vi "Destroy Subscription.vi"(8 "error in (no error)":errorcluster, 11 "Subscription in":refnum<class "Subscription.lvclass">) -> (0 "error out":errorcluster, 3 "Subscription out":refnum<class "Subscription.lvclass">)   [LabVIEW 2013, in "MQTT Server.lvlib" / "Subscription.lvclass"]
uses:
  Subscription.lvclass
  Subscription.lvclass/Subscription.ctl
  TopicFilter/TopicFilter.lvclass
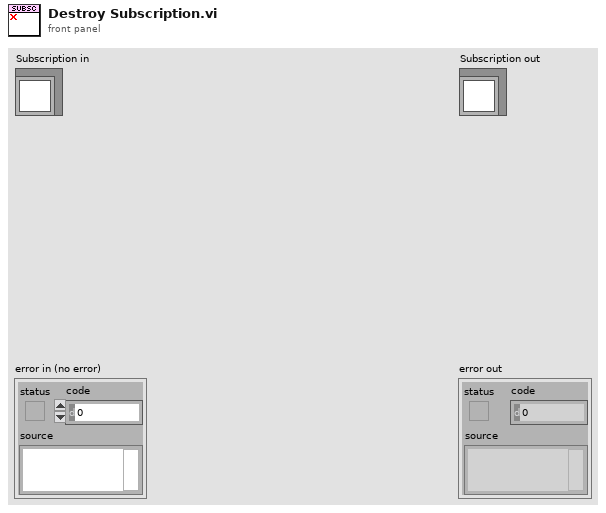
[diagram p1: front panel]
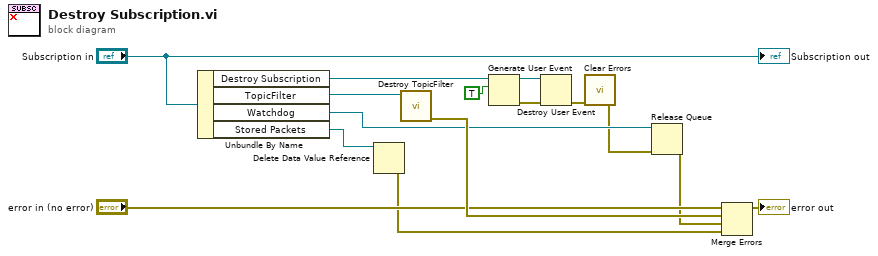
[diagram p0: block diagram]
diagram:
  n1 = Unbundle By Name("Subscription in") -> ("Destroy Subscription"=w10:refnum<user-event>, "TopicFilter"=w14:refnum<class "TopicFilter.lvclass">, "Watchdog"=w5:refnum<queue>, "Stored Packets"=w2:refnum<data-value>)
  n2 = Delete Data Value Reference(data value reference=w2) -> (error out=w1:errorcluster)  [unwired: 1 in, 1 out]
  n3 = call "Destroy TopicFilter.vi"("TopicFilter in"=w14) -> ("error out"=w13:errorcluster)  [unwired: 9 in, 1 out]
  n4 = Generate User Event(user event=w10, event data cluster=TRUE ("event data")) -> (user event out=w8:refnum<user-event>, error out=w7:errorcluster)  [unwired: 2 in]
  n5 = Destroy User Event(user event=w8, error in=w7) -> (error out=w6:errorcluster)
  n6 = call <vilib>:"Clear Errors.vi"("error in (no error)"=w6) -> ("error out"=w4:errorcluster)  [unwired: 6 in]
  n7 = Release Queue(queue=w5, error in (no error)=w4) -> (error out=w3:errorcluster)  [unwired: 1 in, 2 out]
  n8 = Merge Errors("error in (no error)", w13, w3, w1) -> (→"error out":errorcluster)
  "Subscription out" <- "Subscription in"
